vi "GetDoubleGlobalVariable.vi"(8 "error in (no error)":errorcluster, 10 "varNumber":i32, 11 "controller in":refnum<k24>) -> (0 "error out":errorcluster, 2 "double value out":dbl, 3 "controller out":refnum<k24>)   [LabVIEW 2010]
uses:
  c:/aerotech/controller/5.xx.xxx/A3200/pc/labview/2010/bin/Aerotech.A3200.dll
  bin/Aerotech.A3200.dll
  c:/aerotech/controller/5.xx.xxx/A3200/pc/labview/2010/bin/Aerotech.A3200.LabVIEW.dll
  bin/Aerotech.A3200.LabVIEW.dll
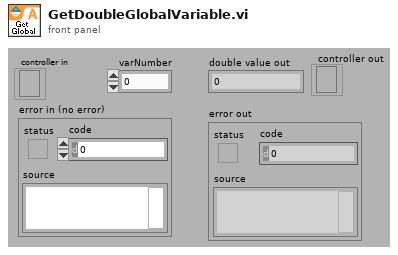
[diagram p1: front panel]
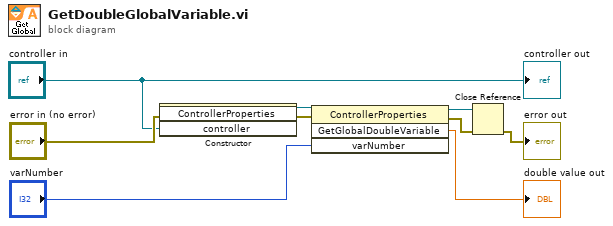
[diagram p0: block diagram]
diagram:
  n1 = constructor class="ControllerProperties"(error in="error in (no error)", "controller"="controller in") -> (reference out=w9:refnum<k24>, error out=w7:errorcluster)  [unwired: 2 in, 2 out]
  n2 = invoke class="ControllerProperties" method="GetGlobalDoubleVariable"(reference=w9, error in=w7, "varNumber"="varNumber") -> (reference out=w3:refnum<k24>, error out=w2:errorcluster, "GetGlobalDoubleVariable"=→"double value out":dbl)  [unwired: 1 in, 1 out]
  n3 = Close Reference(reference=w3, error in (no error)=w2) -> (error out=→"error out":errorcluster)
  "controller out" <- "controller in"
